vi "acquisitionAxisProjection.vi"(1 "axis (z)":u16(ring)=2 items=["x", "y", "z"], 2 "z stack":u16[][][](array[numeric])) -> (0 "projected img":u64[][](array[numeric]))   [LabVIEW 2017]
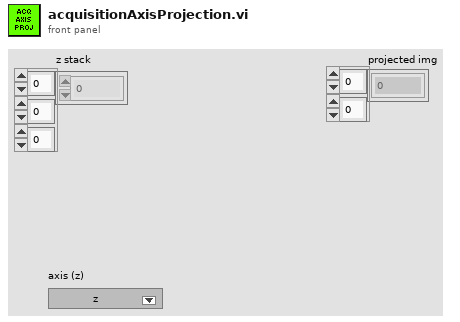
[diagram p1: front panel]
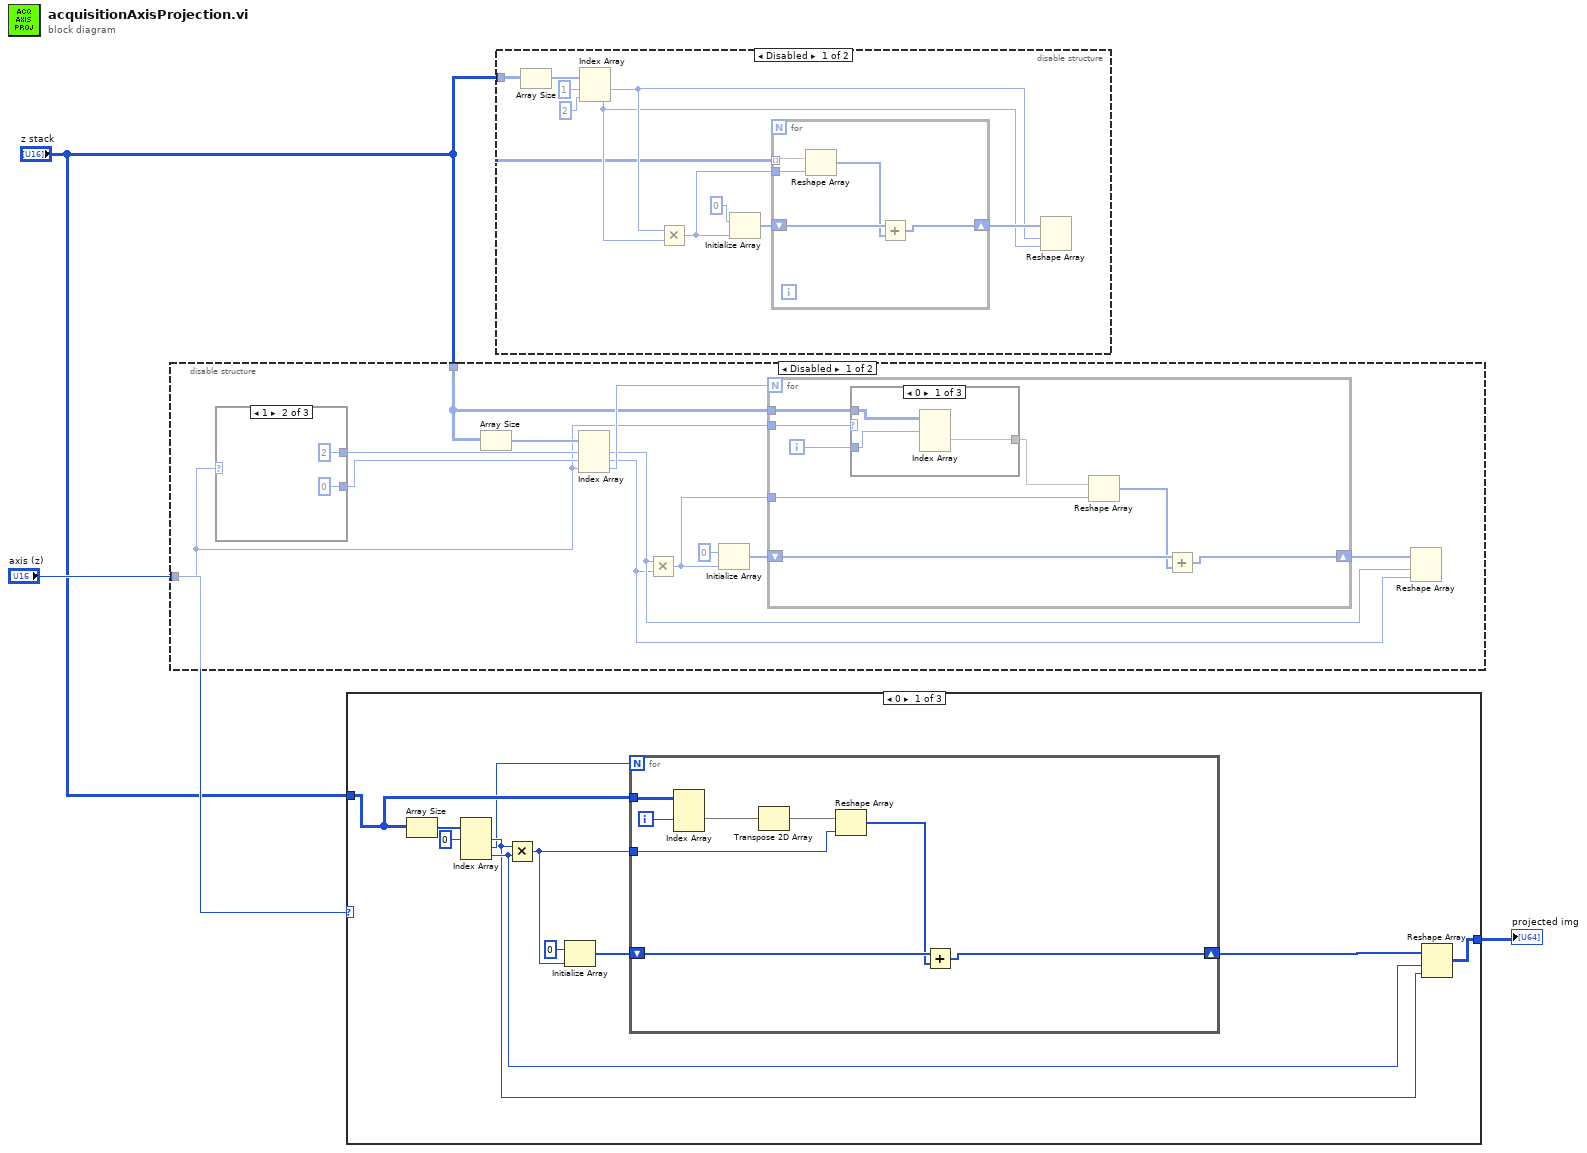
[diagram p0: block diagram]
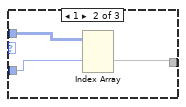
[diagram p2: hidden frame]
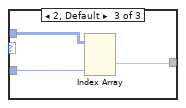
[diagram p3: hidden frame]
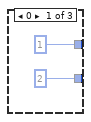
[diagram p4: hidden frame]
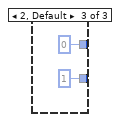
[diagram p5: hidden frame]
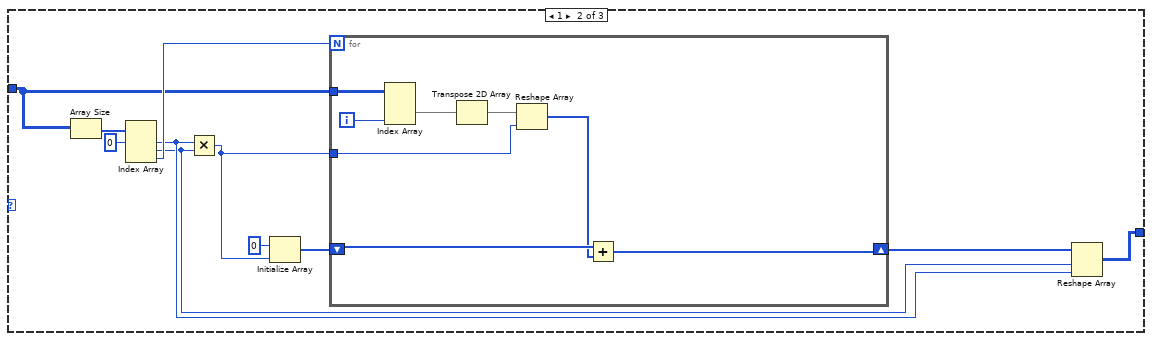
[diagram p7: hidden frame]
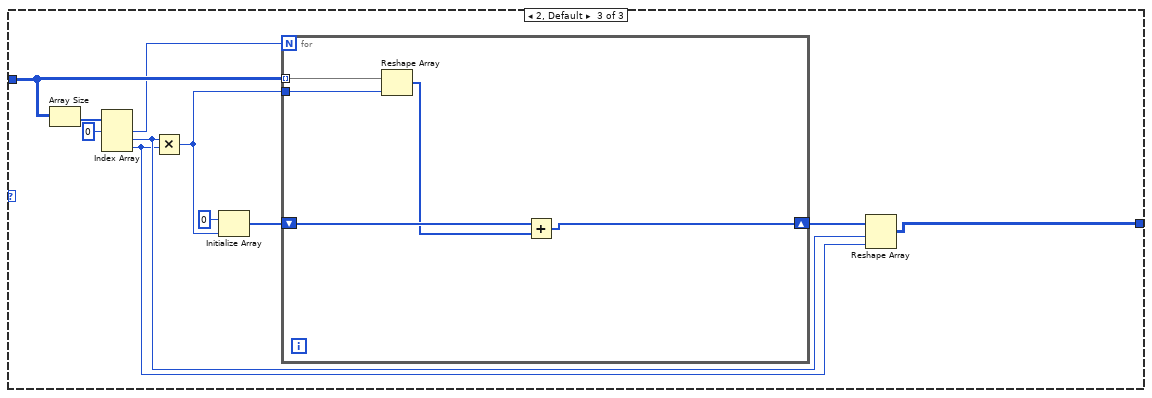
[diagram p8: hidden frame]
diagram:
  n1 = disable-structure shown="Disabled" {
    disable-tunnel: "axis (z)" -> [w5 _]
    disable-tunnel: "z stack" -> [w4 _]
    frame Disabled {
      n2 = case shown="1" w5 {
        tunnel: [1 2 0] -> w14
        tunnel: [2 0 1] -> w13
        frame 0 {
        }
        frame 1 {
        }
        frame 2, Default {
        }
      }
      n3 = Array Size(array=w4) -> (size(s)=w15:i32[])
      n4 = Index Array(array=w15, index #1=w14, index #2=w13, index #3=w5) -> (element #1=w7:i32, element #2=w6:i32, element #3=w11:i32)
      n5 = Multiply(x=w7, y=w6) -> (x*y=w9:i32)
      n6 = Initialize Array(u64 0 ("element"), w9) -> (w10:u64[])
      n7 = for {
        N: w11 -> [_]
        tunnel: w4 -> [w23]
        tunnel: w5 -> [w22]
        shift-right: [w16] -> w8
        shift-left: w10 -> [w20]
        tunnel: w9 -> [w18]
        i -> [w21]
        n8 = case shown="0" w22 {
          tunnel: w23 -> [w26 w29 w31]
          tunnel: w21 -> [w25 w28 w32]
          tunnel: [w24 w27 w30] -> w19
          frame 0 {
            n9 = Index Array(array=w26, index (dim 0)=w25) -> (element=w24:u16[][])  [unwired: 2 in]
          }
          frame 1 {
            n10 = Index Array(array=w29, index (dim 1)=w28) -> (element=w27:u16[][])  [unwired: 2 in]
          }
          frame 2, Default {
            n11 = Index Array(array=w31, index (dim 2)=w32) -> (element=w30:u16[][])  [unwired: 2 in]
          }
        }
        n12 = Reshape Array(w19, w18) -> (w17:u16[])
        n13 = Add(x=w20, y=w17) -> (x+y=w16:u64[])
      }
      n14 = Reshape Array(w8, w7, w6) -> ()  [unwired: 1 out]
    }
    frame Enabled {
    }
  }
  n15 = case shown="0" "axis (z)" {
    tunnel: "z stack" -> [w45 w63 w86]
    tunnel: [w42 w60 w77] -> w1
    frame 0 {
      n16 = Array Size(array=w45) -> (size(s)=w49:i32[])
      n17 = Index Array(array=w49, index #1=0 ("index")) -> (element #1=w43:i32, element #2=w41:i32, element #3=w44:i32)  [unwired: 2 in]
      n18 = Multiply(x=w43, y=w44) -> (x*y=w40:i32)
      n19 = Initialize Array(u64 0 ("element"), w40) -> (w46:u64[])
      n20 = for {
        N: w41 -> [_]
        shift-right: [w52] -> w39
        shift-left: w46 -> [w54]
        tunnel: w45 -> [w57]
        tunnel: w40 -> [w55]
        i -> [w56]
        n21 = Index Array(array=w57, index (dim 1)=w56) -> (element=w51:u16[][])  [unwired: 2 in]
        n22 = Transpose 2D Array(2D array=w51) -> (transposed array=w50:u16[][])
        n23 = Reshape Array(w50, w55) -> (w53:u16[])
        n24 = Add(x=w54, y=w53) -> (x+y=w52:u64[])
      }
      n25 = Reshape Array(w39, w44, w43) -> (w42:u64[][])
    }
    frame 1 {
      n26 = Array Size(array=w63) -> (size(s)=w68:i32[])
      n27 = Index Array(array=w68, index #1=0 ("index")) -> (element #1=w59:i32, element #2=w58:i32, element #3=w65:i32)  [unwired: 2 in]
      n28 = Multiply(x=w59, y=w58) -> (x*y=w62:i32)
      n29 = Initialize Array(u64 0 ("element"), w62) -> (w64:u64[])
      n30 = for {
        N: w65 -> [_]
        shift-right: [w70] -> w61
        shift-left: w64 -> [w72]
        tunnel: w63 -> [w76]
        tunnel: w62 -> [w73]
        i -> [w75]
        n31 = Index Array(array=w76, index (dim 2)=w75) -> (element=w74:u16[][])  [unwired: 2 in]
        n32 = Transpose 2D Array(2D array=w74) -> (transposed array=w69:u16[][])
        n33 = Reshape Array(w69, w73) -> (w71:u16[])
        n34 = Add(x=w72, y=w71) -> (x+y=w70:u64[])
      }
      n35 = Reshape Array(w61, w58, w59) -> (w60:u64[][])
    }
    frame 2, Default {
      n36 = Array Size(array=w86) -> (size(s)=w85:i32[])
      n37 = Index Array(array=w85, index #1=0 ("index")) -> (element #1=w81:i32, element #2=w79:i32, element #3=w78:i32)  [unwired: 2 in]
      n38 = Multiply(x=w79, y=w78) -> (x*y=w82:i32)
      n39 = Initialize Array(u64 0 ("element"), w82) -> (w83:u64[])
      n40 = for {
        N: w81 -> [_]
        tunnel: w86 -> [w92] mode=indexing
        shift-right: [w88] -> w80
        shift-left: w83 -> [w90]
        tunnel: w82 -> [w91]
        n41 = Reshape Array(w92, w91) -> (w89:u16[])
        n42 = Add(x=w90, y=w89) -> (x+y=w88:u64[])
      }
      n43 = Reshape Array(w80, w79, w78) -> (w77:u64[][])
    }
  }
  "projected img" <- w1
  n44 = disable-structure shown="Disabled" {
    disable-tunnel: "z stack" -> [w93 _]
    frame Disabled {
      n45 = Array Size(array=w93) -> (size(s)=w102:i32[])
      n46 = Index Array(array=w102, index #1=1 ("index"), index #2=2 ("index")) -> (element #1=w95:i32, element #2=w94:i32)
      n47 = Multiply(x=w95, y=w94) -> (x*y=w97:i32)
      n48 = Initialize Array(u64 0 ("element"), w97) -> (w98:u64[])
      n49 = for {
        shift-right: [w103] -> w96
        shift-left: w98 -> [w105]
        tunnel: w93 -> [w107] mode=indexing
        tunnel: w97 -> [w106]
        n50 = Reshape Array(w107, w106) -> (w104:u16[])
        n51 = Add(x=w105, y=w104) -> (x+y=w103:u64[])
      }
      n52 = Reshape Array(w96, w95, w94) -> ()  [unwired: 1 out]
    }
    frame Enabled {
    }
  }
